vi "build resource info.vi"(5 "get unmapped?":bool, 6 "datatype":string, 7 "get mapped?":bool, 8 "error in (no error)":errorcluster, 9 "name in bitfile":string, 10 "input type":string, 11 "FPGA CD Ref":T1 format="%.0x") -> (0 "error out":errorcluster, 2 "include?":bool, 3 "visualizer entry":T2 {"FPGA CD Ref" format="%.0x"; "reserver" format="%.0x"})   [LabVIEW 2016, in "FPGA Resource Manager.lvlib"]
uses:
  FPGA Resource Manager.lvlib
  resource info.ctl
  <vilib>/NI Veristand/Custom Device API/Custom Device Item Ref.ctl
  <vilib>/NI VeriStand/Custom Device API/Custom Device API.lvlib
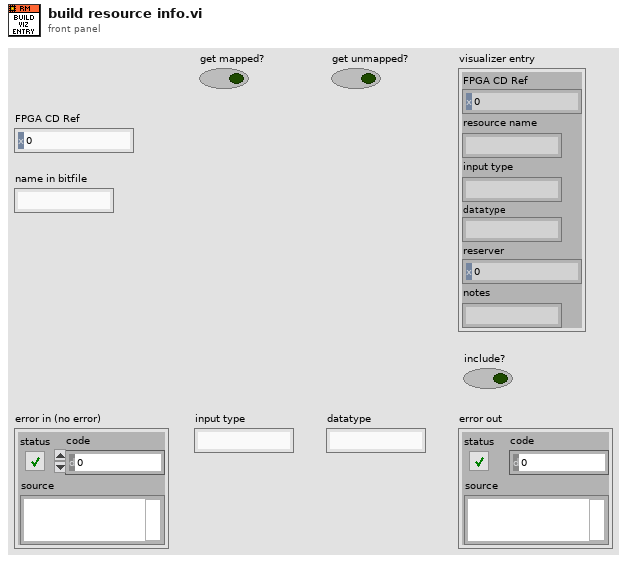
[diagram p1: front panel]
types:
  T1 = typedef "Custom Device API.lvlib/Custom Device Item Ref.ctl" = u64
  T2 = typedef "FPGA Resource Manager.lvlib/resource info.ctl" = cluster{"FPGA CD Ref":T1, "resource name":string, "input type":string, "datatype":string, "reserver":T1, "notes":string}
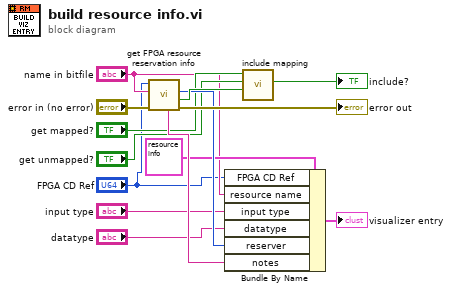
[diagram p0: block diagram]
diagram:
  n1 = call "get FPGA resource reservation info.vi"("error in (no error)"="error in (no error)", "Name in Bitfile"="name in bitfile", "Item Ref in"="FPGA CD Ref") -> ("error out"=→"error out":errorcluster, "found?"=w12:bool, "Reserver Node Ref"=w10:T1, "notes"=w11:string)  [unwired: 4 in, 1 out]
  n2 = Bundle By Name(cluster=T2 {"FPGA CD Ref"=18446744073709551615, "resource name"="", "input type"="", "datatype"="", "reserver"=18446744073709551615, "notes"=""} ("visualizer entry"), "FPGA CD Ref"="FPGA CD Ref", "resource name"="name in bitfile", "input type"="input type", "datatype"="datatype", "reserver"=w10, "notes"=w11) -> (→"visualizer entry":T2)
  n3 = call "include mapping.vi"("is mapped?"=w12, "get unmapped?"="get unmapped?", "get mapped?"="get mapped?") -> ("include?"=→"include?":bool)  [unwired: 8 in]
